vi "Lockin.DAQ.GetPrivateEvents.vi"(8 "error in (no error)":errorcluster, 11 "Lockin.DAQ":refnum<class "Lockin.DAQ.lvclass">) -> (0 "error out":errorcluster, 2 "Private Events":T1, 3 "Lockin.DAQ":refnum<class "Lockin.DAQ.lvclass">)   [LabVIEW 2016, in "Lockin.DAQ.lvclass"]
doc: "---------------------------------------------------------------\nJKI State Machine Objects™\nhttp://jki.net/state-machine-objects/\nCopyright (C) 2005-2015, JKI <info@jki.net>\nALL RIGHTS RESERVEDJKI State Machine Objects (SMO) 1.0.0.4\nJKI - JKI\nCopyright (c) 2015, JKI"
uses:
  Lockin.DAQ.lvclass
  Typedefs/PrivateEvents--Cluster.ctl
  Typedefs/PrivateEvents--Lockin.DAQ.setAOconfig.ctl
  Typedefs/AO.config-array.ctl
  Typedefs/AO.config-cluster.ctl
  Typedefs/446xAO-enum.ctl
  Typedefs/DAQType-enum.ctl
  Typedefs/PrivateEvents--Lockin.DAQ.setAIconfig.ctl
  Typedefs/AI.config-array.ctl
  Typedefs/AI.config-cluster.ctl
  Typedefs/AI.coupling-enum.ctl
  Typedefs/446xAI-enum.ctl
  Typedefs/AI Simulation-enum.ctl
  Typedefs/PrivateEvents--Lockin.DAQ.setAO.ctl
  Typedefs/AO-cluster.ctl
  Instrument.Lockinl.UI/Typedefs/AO Channel--Cluster.ctl
  Typedefs/Function-enum.ctl
  Typedefs/PrivateEvents--Lockin.DAQ.setREF.ctl
  Typedefs/REF-cluster.ctl
  Instrument.Lockinl.UI/Typedefs/REF Channel--Cluster.ctl
  Typedefs/PrivateEvents--Lockin.DAQ.setSampling.ctl
  Typedefs/Sampling.ctl
  Typedefs/Sample Mode--Ring.ctl
  Typedefs/PrivateEvents--Lockin.DAQ.setState.ctl
  Typedefs/Set State-enum.ctl
  Typedefs/PrivateEvents--Lockin.DAQ.setInputGain.ctl
  Typedefs/PrivateEvents--Lockin.DAQ.setSweep.ctl
  Typedefs/Sweep Configuration--Cluster.ctl
  Instrument.Lockinl.UI/Typedefs/Sweep Channel--Cluster.ctl
  Typedefs/Sweep Pattern--Enum.ctl
  Typedefs/PrivateEvents--Lockin.DAQ.measureOffset.ctl
  Typedefs/PrivateEvents--Lockin.DAQ.zeroOffset.ctl
  Typedefs/PrivateEvents--Lockin.DAQ.setPreFilter.ctl
  Typedefs/AI Prefilter-cluster.ctl
  Typedefs/PrivateEvents--Lockin.DAQ.autoContigureDAQ.ctl
  Typedefs/PrivateEvents--LockinDAQ.setCalibration.ctl
  Typedefs/PrivateEvents--Lockin.DAQ.setAI.ctl
  Typedefs/AI-cluster.ctl
  Instrument.Lockinl.UI/Typedefs/AI Channel--Cluster.ctl
  Lockin.DAQ.lvclass/Lockin.DAQ.ctl
  Instrument.Lockinl.UI/Instrument.Lockin.UI.lvclass
panel:
  # "For instructions on how to use the JKI State Machine Objects, examples and video tutorials, visit:\nhttp://jki.net/state-machine-objects/\n\nJKI State Machine Objects™\nhttp://jki.net/state-machine-objects/\nCopyright (C) 2005-2015, JKI <info@jki.net>\nALL RIGHTS RESERVED"
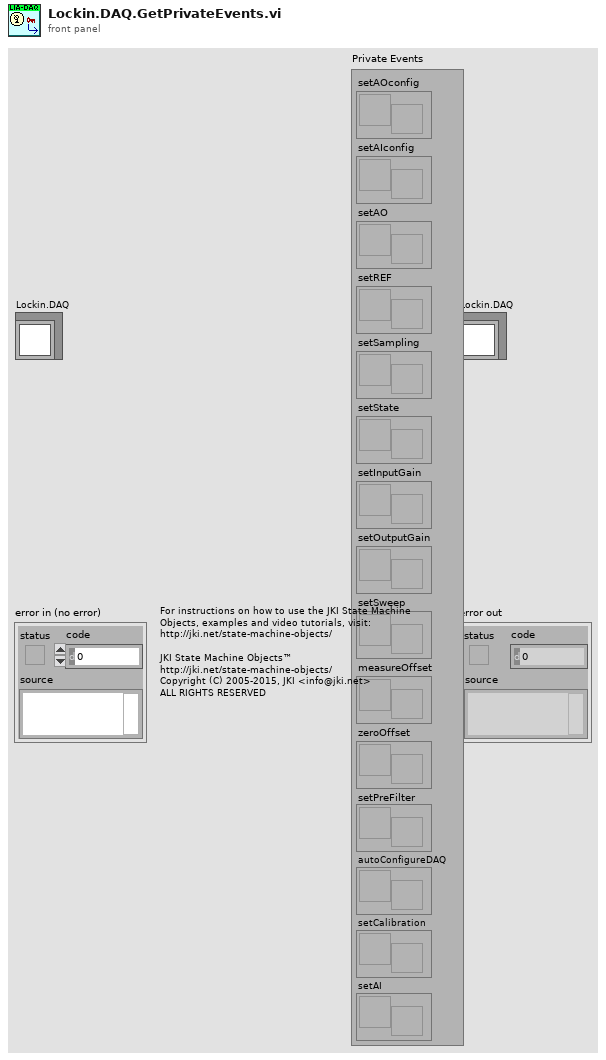
[diagram p1: front panel]
types:
  T1 = typedef "Lockin.DAQ.lvclass/PrivateEvents--Cluster.ctl" = cluster{"setAOconfig":refnum<user-event>, "setAIconfig":refnum<user-event>, "setAO":refnum<user-event>, "setREF":refnum<user-event>, "setSampling":refnum<user-event>, "setState":refnum<user-event>, "setInputGain":refnum<user-event>, "setOutputGain":refnum<user-event>, "setSweep":refnum<user-event>, "measureOffset":refnum<user-event>, "zeroOffset":refnum<user-event>, "setPreFilter":refnum<user-event>, "autoConfigureDAQ":refnum<user-event>, "setCalibration":refnum<user-event>, "setAI":refnum<user-event>}
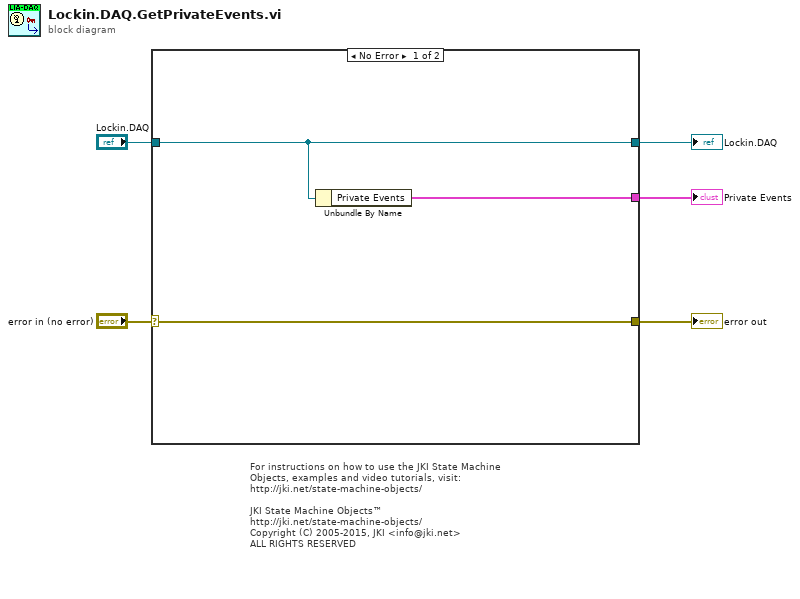
[diagram p0: block diagram]
diagram:
  # "For instructions on how to use the JKI State Machine Objects, examples and video tutorials, visit:\nhttp://jki.net/state-machine-objects/\n\nJKI State Machine Objects™\nhttp://jki.net/state-machine-objects/\nCopyright (C) 2005-2015, JKI <info@jki.net>\nALL RIGHTS RESERVED"
  n1 = case shown="No Error" "error in (no error)" {
    selector: "error in (no error)" -> [w7 w9]
    tunnel: "Lockin.DAQ" -> [w6 w10]
    tunnel: [w7 w9] -> w4
    tunnel: [w6 w10] -> w3
    tunnel: [w8 _] -> w1
    frame No Error {
      n2 = Unbundle By Name(w6) -> ("Private Events"=w8:T1)
    }
    frame Error {
    }
  }
  "error out" <- w4
  "Lockin.DAQ" <- w3
  "Private Events" <- w1
